vi "BRig_Host_comm_tcp_connect_HOSTwrite.vi"(8 "input_error":errorcluster, 10 "input_connected":bool, 11 "input_hTCP":refnum<k5>) -> (0 "output_error":errorcluster, 2 "output_connected":bool, 3 "output_hTCP":refnum<k5>, 4 "output_Twait":u32)   [LabVIEW 2014]
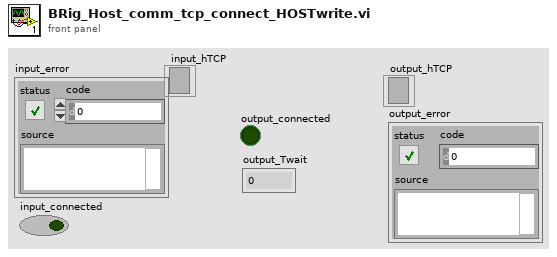
[diagram p1: front panel]
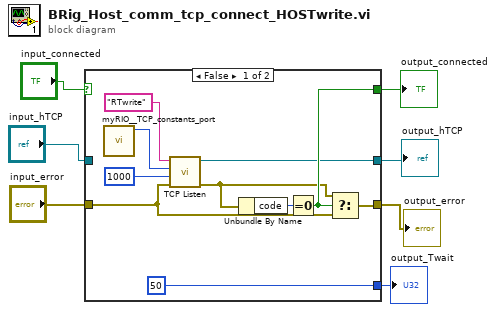
[diagram p0: block diagram]
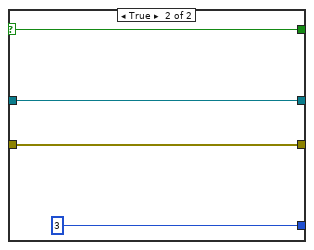
[diagram p2: hidden frame]
diagram:
  n1 = case shown="False" "input_connected" {
    selector: "input_connected" -> [_ w21]
    tunnel: [w16 w21] -> w7
    tunnel: [w15 w20] -> w6
    tunnel: "input_error" -> [w14 w20]
    tunnel: [w10 w19] -> w3
    tunnel: "input_hTCP" -> [_ w19]
    tunnel: [u32 50 ("milliseconds to wait") u32 3 ("milliseconds to wait")] -> w1
    frame False {
      n2 = call "myRIO__TCP_constants_port.vi"() -> ("output_TCP_port"=w12:u16)  [unwired: 11 in]
      n3 = call <vilib>:"TCP Listen.vi"("error in (no error)"=w14, "timeout ms (wait forever: -1)"=1000, "port"=w12, "service name"="RTwrite") -> ("error out"=w13:errorcluster, "connection ID"=w10:refnum<k5>)  [unwired: 3 in, 3 out]
      n4 = Unbundle By Name(w13) -> ("code"=w17:i32)
      n5 = Equal To 0?(x=w17) -> (x = 0?=w16:bool)
      n6 = Select(t=w13, s=w16, f=w14) -> (s? t:f=w15:errorcluster)
    }
    frame True {
    }
  }
  "output_error" <- w6
  "output_connected" <- w7
  "output_hTCP" <- w3
  "output_Twait" <- w1
